vi "Example IMAQdx Cam and XDisplay.vi"() -> ()   [LabVIEW 2009]
uses:
  <vilib>/userDefined/High Color/IMAQdx.ctl
  XDisplay/POLARIS IMAQ Display.xctl
  IMAQdx Cam/IMAQdx Cam.lvclass
  Analyze Classes/Analyze Fluence/Analyze Fluence.lvclass
  Analyze Classes/Analyze Q-Factor/Analyze q-Factor.lvclass
  Analyze Classes/Analyze Distanz/Analyze Distanz.lvclass
panel:
  in  "Energy":dbl[unit]
  in  "WorkDir":path
  in  "ConfigDir":path
  in  "XDisplay":cluster{"Image":T1}(xcontrol)
  in  "stop":bool
  in  "Camera Name":T2="JustageCam"
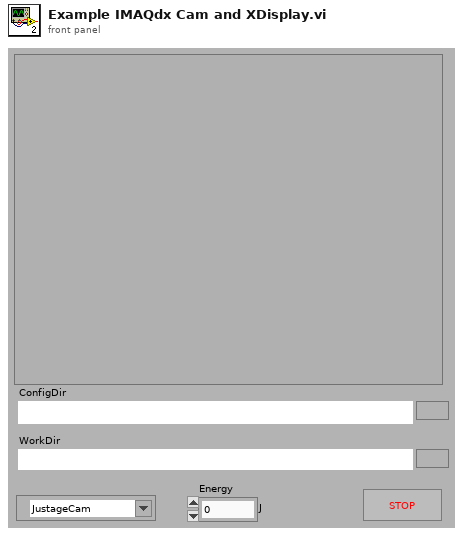
[diagram p1: front panel]
types:
  T1 = typedef "IMAQ Image.ctl" = refnum<image>
  T2 = typedef "IMAQdx.ctl" = refnum<k21>
  T3 = cluster{"Desired Font (Application)":enum16{"User-specified Font", "Application Font", "System Font", "Dialog Font"}, "[User-specified Font]":cluster{"Font Name":string, "Size":i16, "Strikeout?":bool, "Italic?":bool, "Underline?":bool, "Outline?":bool, "Shadow?":bool, "Bold?":bool, "Rotation Angle":dbl}, "Horizontal Alignment":i16, "Vertical Alignment":i16}
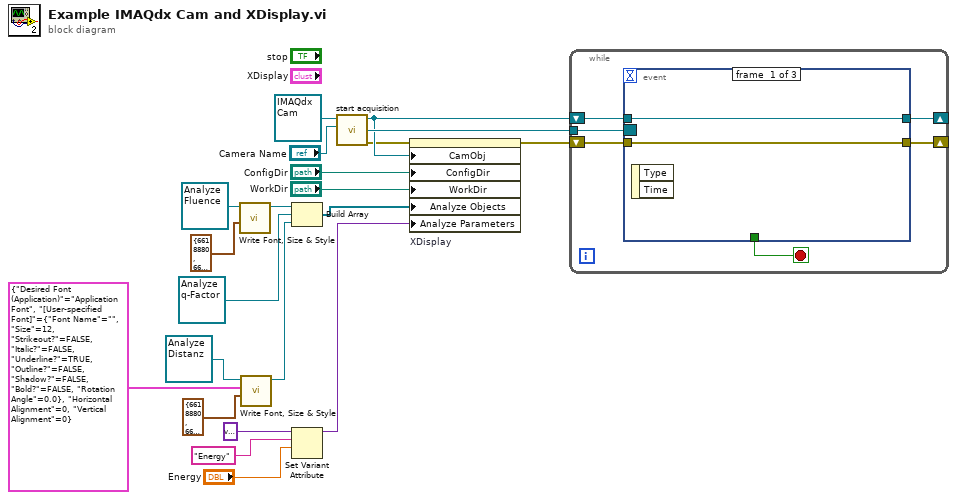
[diagram p0: block diagram]
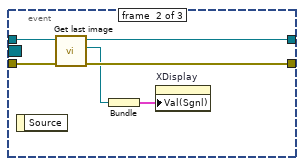
[diagram p2: hidden frame]
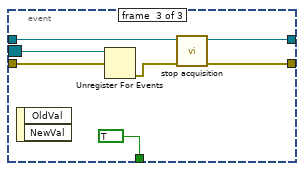
[diagram p3: hidden frame]
diagram:
  n1 = call-dynamic "Write Font, Size & Style.vi"("Overlay colors"=cluster{"Border":u32, "Text":u32} {"Border"=6618880, "Text"=6618880}, "Analyze BaseClass in"=refnum<class "Analyze Fluence.lvclass"> refnum ("Analyze.lvlib:Analyze Fluence.lvclass")) -> ("Analyze BaseClass out"=w6:refnum<class "Analyze Fluence.lvclass">)  [unwired: 8 in, 1 out]
  n2 = call-dynamic "Write Font, Size & Style.vi"("Overlay colors"=cluster{"Border":u32, "Text":u32} {"Border"=6618880, "Text"=6618880}, "Font, Size & Style"=T3 {"Desired Font (Application)"=enum."Application Font", "[User-specified Font]"={"Font Name"="", "Size"=12, "Strikeout?"=FALSE, "Italic?"=FALSE, "Underline?"=TRUE, "Outline?"=FALSE, "Shadow?"=FALSE, "Bold?"=FALSE, "Rotation Angle"=0.0}, "Horizontal Alignment"=0, "Vertical Alignment"=0}, "Analyze BaseClass in"=refnum<class "Analyze Distanz.lvclass"> refnum ("Analyze.lvlib:Analyze Distanz.lvclass")) -> ("Analyze BaseClass out"=w3:refnum<class "Analyze Distanz.lvclass">)  [unwired: 7 in, 1 out]
  n3 = Build Array(w6, refnum<class "Analyze q-Factor.lvclass"> refnum ("Analyze.lvlib:Analyze q-Factor.lvclass"), w3) -> (w12:refnum<class "Analyze BaseClass.lvclass">[])
  n4 = Set Variant Attribute(Variant=variant ("Analyze Parameters"), name="Energy", value="Energy") -> (Variant out=w10:variant)  [unwired: 1 in, 2 out]
  n5 = call-dynamic "start acquisition.vi"("Camera Name"="Camera Name", "IMAQdx Cam in"=refnum<class "IMAQdx Cam.lvclass"> refnum ("IMAQdx Cam.lvclass")) -> ("error out"=w17:errorcluster, "Event Registration Refnum"=w20:refnum<event-registration>, "IMAQdx Cam out"=w18:refnum<class "IMAQdx Cam.lvclass">)  [unwired: 7 in]
  n6 = property on="XDisplay" class="POLARIS IMAQ Display (strict)"(error in=w17, "CamObj"=w18, "ConfigDir"="ConfigDir", "WorkDir"="WorkDir", "Analyze Objects"=w12, "Analyze Parameters"=w10) -> (error out=w16:errorcluster)  [unwired: 1 in, 1 out]
  n7 = while {
    tunnel: w20 -> [w22]
    shift-right: [w25] -> _
    shift-left: w18 -> [w27]
    shift-right: [w24] -> _
    shift-left: w16 -> [w26]
    stop <- w23 stop-if-true
    n8 = event shown="[1] <Session Out>: FrameDone" {
      selector: w22 -> [_ _ w41]
      dyn-events: _ -> [_ _ _]
      timeout: _ -> [_ _ _]
      tunnel: w27 -> [w28 w35 w39]
      tunnel: w26 -> [w29 w34 w40]
      tunnel: [w28 w33 w37] -> w25
      tunnel: [w29 w32 w36] -> w24
      tunnel: [_ _ TRUE] -> w23
      event #0 {
        n9 = event-data() -> ()  [unwired: 1 in, 2 out]
      }
      event #1 {
        n10 = event-data() -> ()  [unwired: 1 in, 1 out]
        n11 = call-dynamic "Get last image.vi"("error in (no error)"=w34, "IMAQdx Cam in"=w35) -> ("error out"=w32:errorcluster, "Image Out"=w31:T1, "IMAQdx Cam out"=w33:refnum<class "IMAQdx Cam.lvclass">)  [unwired: 7 in]
        n12 = Bundle("Image Out"=w31) -> (w30:cluster{"Image Out":T1})  [unwired: 1 in]
        n13 = property on="XDisplay" class="POLARIS IMAQ Display (strict)"("Val(Sgnl)"=w30) -> ()  [unwired: 2 in, 2 out]
      }
      event #2 {
        n14 = event-data() -> ()  [unwired: 1 in, 2 out]
        n15 = Unregister For Events(event registration refnum=w41, error in=w40) -> (error out=w38:errorcluster)
        n16 = call-dynamic "stop acquisition.vi"("error in (no error)"=w38, "IMAQdx Cam in"=w39) -> ("error out"=w36:errorcluster, "IMAQdx Cam out"=w37:refnum<class "IMAQdx Cam.lvclass">)  [unwired: 8 in]
      }
    }
  }
